vi "Grid_Create_Files_Headers.vi"(7 "resume":T1, 8 "Error in (no error)":errorcluster, 9 "Settings":T3={"Drift Correction Settings"={"Drift Correction every"=80, "Drift correction Pixels"=256, "Channel index (0-23)"=0, "MaxImagesBack"=2, "Threshold"=2, "Increment"=8, "max applied Drift Correction"=20, "Correct Drift"=TRUE, "Correlate"=0, "Correct z drift"=FALSE, "zdrift \nDuration (s)"=0.0}, "Spectroscopy Setting"={"Imaging Current"=1e-11, "ref Current"=7e-11, "tip Speed (m/s)"=2e-09, "Imaging Bias"=0.02, "ref Bias"=-0.1, "preSTS delay [ms]"=500, "STS z offset"=2e-10, "during Spec Bias (V)"=-0.1, "trigger1 < Hz"=0.0, "trigger 2 >Hz"=0.0, "autoStop"=FALSE, "Spectroscopy"=0, "PLL ON/OFF"=TRUE, "readjust setpoint every "=1, "z Reference"=FALSE, "Lock In"=TRUE}, "Misc"={"File name"="symmetric_node_zOff=200p", "Email when finished"="cornelius.krull@monash.edu,Dhaneesh.Gopalakrishnan@monash.edu,marina.castelli@monash.edu"}, "Grid Settings"={"type"=1, "type order"=1, "X pixel"=0, "Y pixel"=0, "Grid_Parms"={"center X (m)"=0.0, "center Y (m)"=0.0, "width (m)"=0.0, "height (m)"=0.0, "angle (deg)"=0.0}}} {"Grid Settings"."type order" items=["Line", "Grid"]; "Grid Settings"."type" items=["Line", "Grid"]; "Spectroscopy Setting"."Spectroscopy" items=["Bias", "zSpec"]; "Spectroscopy Setting"."trigger 2 >Hz" format="%#_6p"; "Spectroscopy Setting"."trigger1 < Hz" format="%#_6p"; "Spectroscopy Setting"."during Spec Bias (V)" format="%#_5p"; "Spectroscopy Setting"."STS z offset" format="%#_6p"; "Spectroscopy Setting"."ref Bias" format="%#_6p"; "Spectroscopy Setting"."Imaging Bias" format="%#_6p"; "Spectroscopy Setting"."tip Speed (m/s)" format="%.2p"; "Spectroscopy Setting"."ref Current" format="%#_6p"; "Spectroscopy Setting"."Imaging Current" format="%#_6p"; "Drift Correction Settings"."Correlate" items=["first Frame", "successive Frames"]; "Drift Correction Settings"."max applied Drift Correction" min=1 max=100 step=1 format="%.0p"; "Drift Correction Settings"."Threshold" min=1 step=1; "Drift Correction Settings"."Channel index (0-23)" items=["Current"=0, "Z (m)"=14]}, 11 "Application ref in":refnum<vi>) -> (0 "error out":errorcluster, 1 "topoFilePath":path, 2 "FileRefs":T2, 3 "Application ref out":refnum<vi>)   [LabVIEW 2014]
uses:
  <userlib>/Nanonis Prog Interface V5/Nanonis Prog Interface.lvlib
panel:
  in  "Attributes in":string[][](table)
  # "z Spectroscopy"
  # "GRID points"
  # "Increase this if no Drift was detected for \na certain number of images"
  # "% of image size"
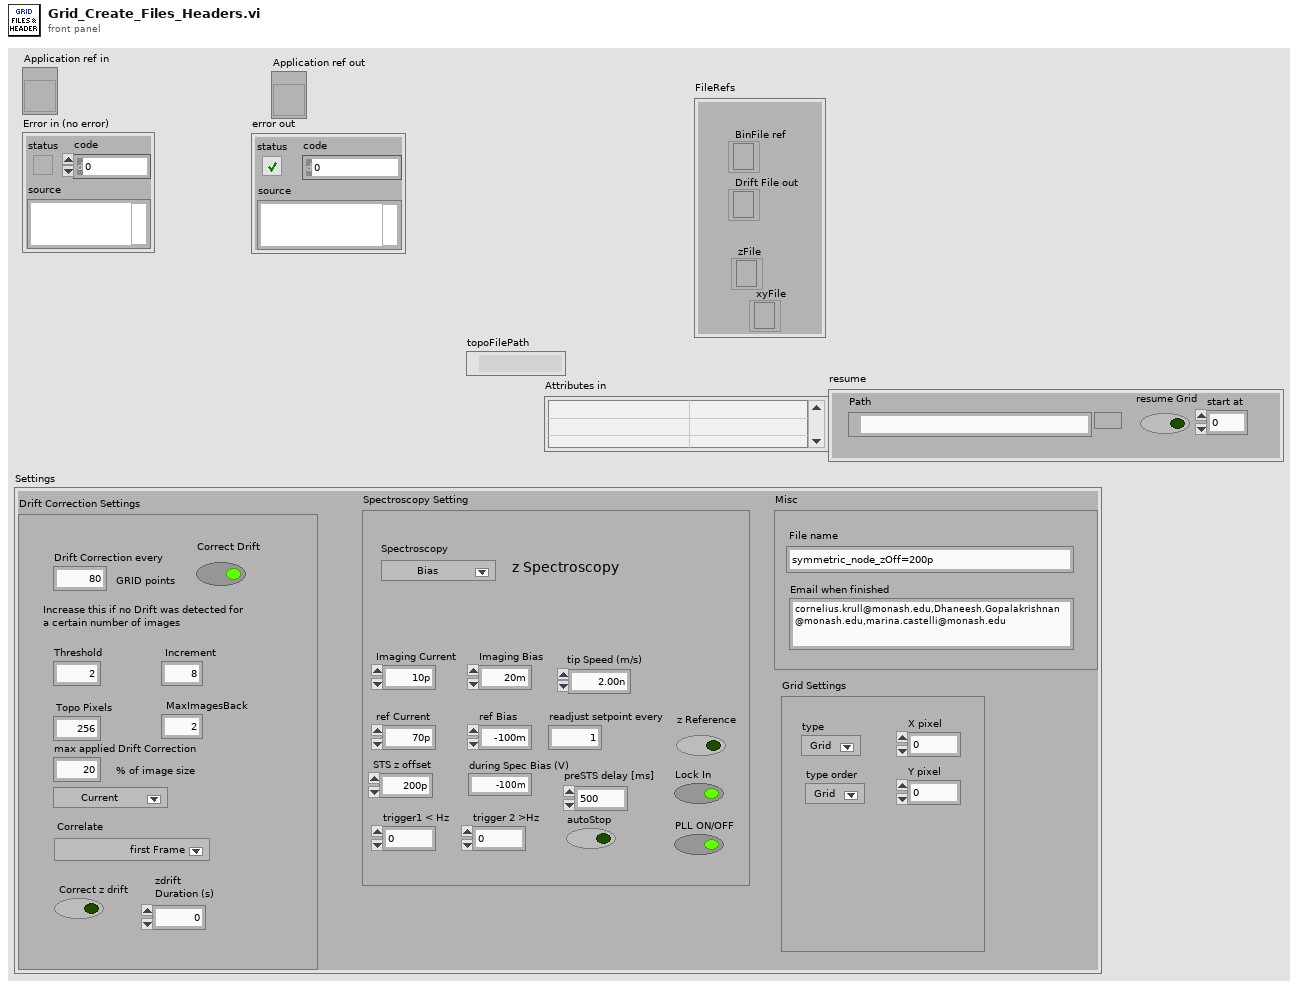
[diagram p1: front panel]
types:
  T1 = cluster{"resume Grid":bool, "Path":path, "start at":i32}
  T2 = cluster{"Drift File out":refnum<file>, "zFile":refnum<file>, "BinFile ref":refnum<file>, "xyFile":refnum<file>}
  T3 = cluster{"Drift Correction Settings":cluster{"Drift Correction every":i32, "Drift correction Pixels":i32, "Channel index (0-23)":u8, "MaxImagesBack":i32, "Threshold":i32, "Increment":i32, "max applied Drift Correction":i32, "Correct Drift":bool, "Correlate":u16, "Correct z drift":bool, "zdrift \nDuration (s)":dbl}, "Spectroscopy Setting":cluster{"Imaging Current":dbl, "ref Current":dbl, "tip Speed (m/s)":sgl, "Imaging Bias":dbl, "ref Bias":dbl, "preSTS delay [ms]":u32, "STS z offset":dbl, "during Spec Bias (V)":sgl, "trigger1 < Hz":sgl, "trigger 2 >Hz":sgl, "autoStop":bool, "Spectroscopy":u16, "PLL ON/OFF":bool, "readjust setpoint every ":i32, "z Reference":bool, "Lock In":bool}, "Misc":cluster{"File name":string, "Email when finished":string}, "Grid Settings":cluster{"type":u16, "type order":u16, "X pixel":i64, "Y pixel":i64, "Grid_Parms":cluster{"center X (m)":sgl, "center Y (m)":sgl, "width (m)":sgl, "height (m)":sgl, "angle (deg)":sgl}}}
  T4 = cluster{"Z averaging time (s)":sgl, "Z offset (m)":sgl, "Initial settling time (s)":sgl}
  T5 = enum16{"open", "replace", "create", "open or create", "replace or create", "replace or create with confirmation"}
  T6 = cluster{"center X (m)":sgl, "center Y (m)":sgl, "width (m)":sgl, "height (m)":sgl, "angle (deg)":sgl}
  T7 = cluster{"Max. slew rate (V/s)":sgl, "Settling time (s)":sgl, "Integration time (s)":sgl}
  T8 = cluster{"End settling time (s)":sgl, "Z control time (s)":sgl}
  T9 = cluster{"Z averaging time (s)":sgl, "Initial settling time (s)":sgl}
  T10 = cluster{"Max. slew rate (m/s)":sgl, "Settling time (s)":sgl, "Integration time (s)":sgl}
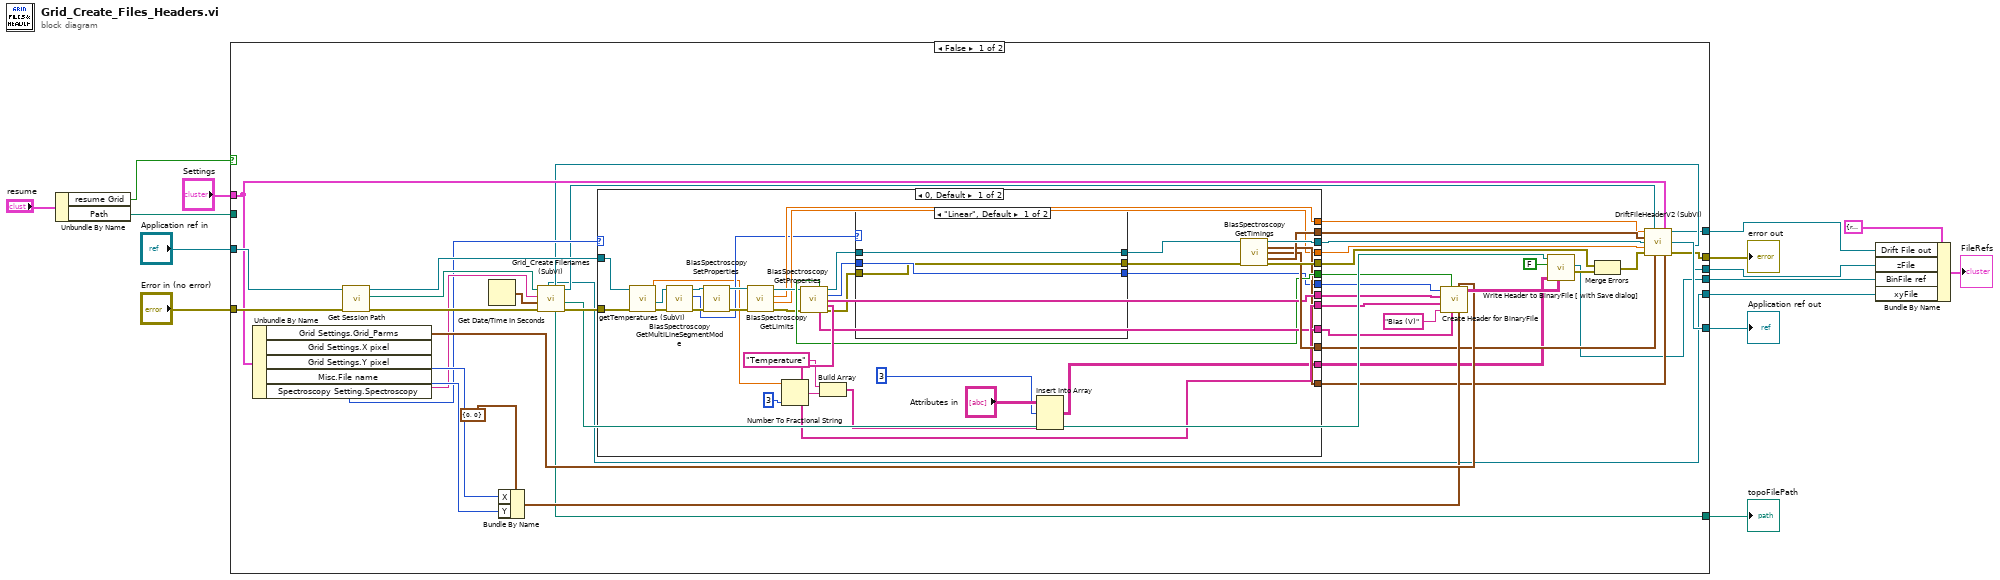
[diagram p0: block diagram]
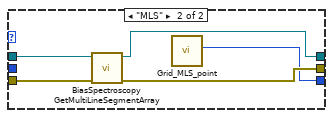
[diagram p2: hidden frame]
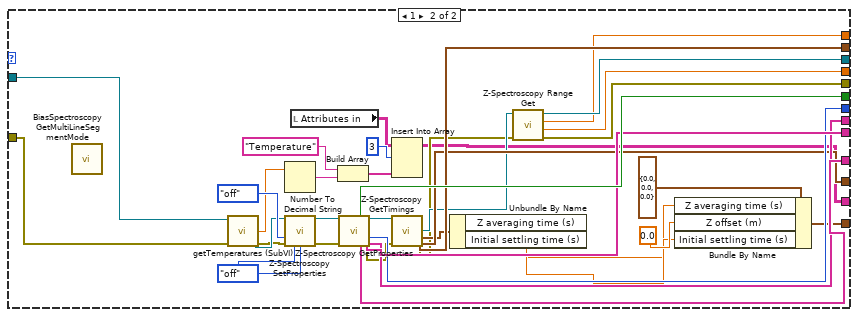
[diagram p3: hidden frame]
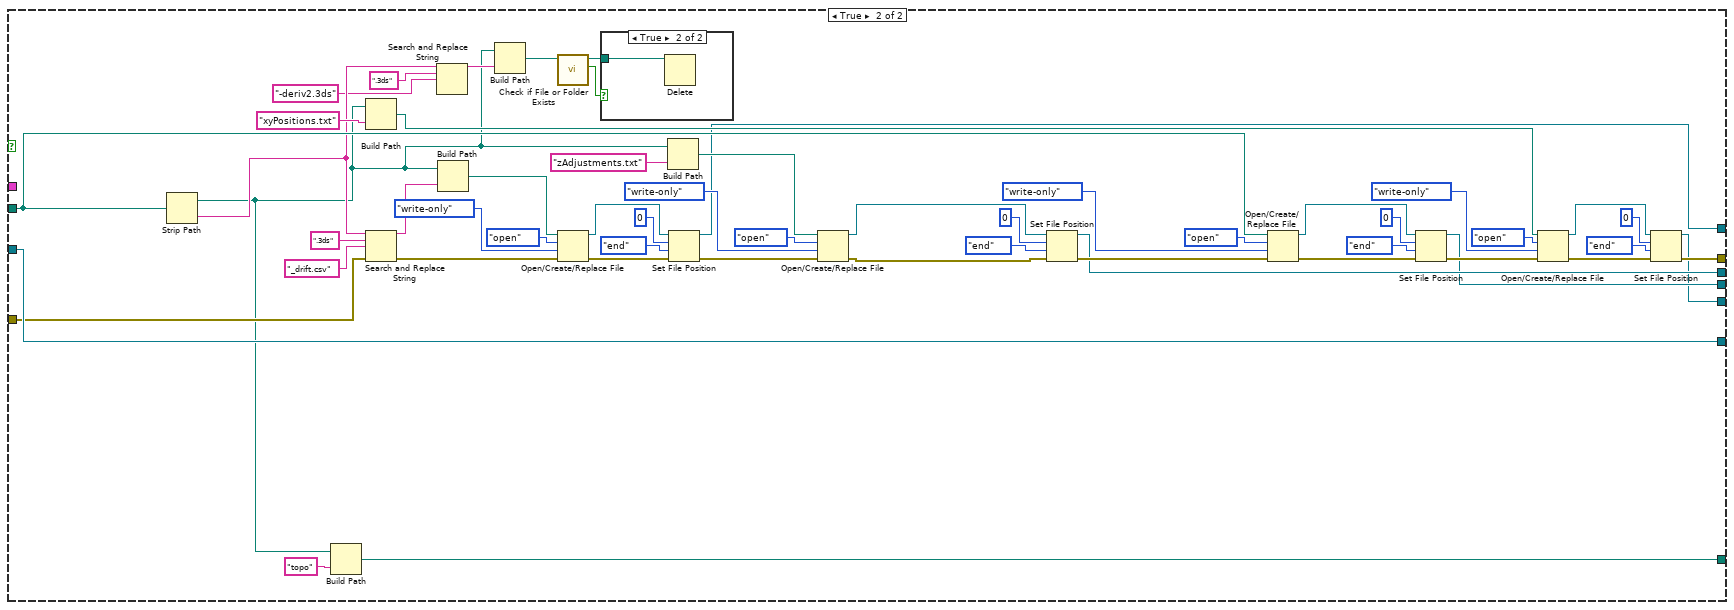
[diagram p4: hidden frame]
diagram:
  n1 = Unbundle By Name("resume") -> ("resume Grid"=w3:bool, "Path"=w1:path)
  n2 = case shown="False" w3 {
    tunnel: "Application ref in" -> [w56 w191]
    tunnel: "Error in (no error)" -> [w55 w170]
    tunnel: "Settings" -> [w32 _]
    tunnel: [w27 w191] -> w12
    tunnel: [w25 w153] -> w11
    tunnel: [w22 w149] -> w10
    tunnel: [w21 w150] -> w9
    tunnel: [w20 w159] -> w8
    tunnel: [w18 w146] -> w5
    tunnel: [w17 w186] -> w2
    tunnel: w1 -> [_ w188]
    frame False {
      n3 = Unbundle By Name(w32) -> ("Grid Settings.Grid_Parms"=w40:T6, "Grid Settings.X pixel"=w38:i64, "Grid Settings.Y pixel"=w37:i64, "Misc.File name"=w31:string, "Spectroscopy Setting.Spectroscopy"=w30:u16)
      n4 = call <userlib>:"Get Session Path.vi"("error in (no error)"=w55, "Application ref in"=w56) -> ("error out"=w53:errorcluster, "Session path"=w54:path, "Application ref out"=w52:refnum<vi>)  [unwired: 7 in]
      n5 = Get Date/Time In Seconds() -> (seconds since 1Jan1904=w19:timestamp)
      n6 = Bundle By Name(cluster=cluster{"X":i32, "Y":i32} {"X"=0, "Y"=0} ("Grid points"), "X"=w38, "Y"=w37) -> (w36:cluster{"X":i32, "Y":i32})
      n7 = call "Grid_Create Filenames (SubVI).vi"("error in (no error)"=w53, "seconds since 1Jan1904"=w19, "File name"=w31, "Session path"=w54) -> ("error out"=w57:errorcluster, "binFilePath"=w50:path, "Drift File out"=w29:refnum<file>, "topoFilePath"=w17:path, "zFile"=w21:refnum<file>, "xyFile"=w18:refnum<file>)  [unwired: 1 in, 1 out]
      n8 = case shown="0, Default" w30 {
        tunnel: [w86 w137] -> w41
        tunnel: [w88 w136] -> w44
        tunnel: [w92 w116] -> w47
        tunnel: [w87 w135] -> w45
        tunnel: [w75 w134] -> w42
        tunnel: [w89 w133] -> w43
        tunnel: w52 -> [w67 w112]
        tunnel: [w91 w131] -> w33
        tunnel: [w90 w130] -> w34
        tunnel: [w85 w119] -> w35
        tunnel: [w93 w117] -> w28
        tunnel: w57 -> [w69 w110]
        tunnel: [w80 w114] -> w24
        tunnel: [w79 w113] -> w23
        tunnel: [w62 w102] -> w16
        frame 0, Default {
          n9 = call "getTemperatures (SubVI).vi"("error in (no error)"=w69, "Application in"=w67) -> ("error out"=w68:errorcluster, "Application ref out"=w66:refnum<vi>, "TSTM"=w65:dbl)  [unwired: 6 in, 1 out]
          n10 = call <userlib>:"BiasSpectroscopy GetMultiLineSegmentMode.vi"("Error in (no error)"=w68, "Application ref in"=w66) -> ("Error out"=w77:errorcluster, "Sweep mode"=w74:enum16{"Linear", "MLS"}, "Application ref out"=w78:refnum<vi>)  [unwired: 5 in]
          n11 = call <userlib>:"BiasSpectroscopy SetProperties.vi"("Application ref in"=w78, "Error in (no error)"=w77) -> ("Application ref out"=w84:refnum<vi>, "Error out"=w81:errorcluster)  [unwired: 12 in]
          n12 = call <userlib>:"BiasSpectroscopy GetLimits.vi"("Error in (no error)"=w81, "Application ref in"=w84) -> ("Error out"=w82:errorcluster, "End value (V)"=w79:sgl, "Start value (V)"=w80:sgl, "Application ref out"=w83:refnum<vi>)  [unwired: 4 in]
          n13 = Number To Fractional String(number=w65, precision (6)=i16 3 ("width (-)")) -> (F-format string=w60:string)  [unwired: 2 in]
          n14 = call <userlib>:"BiasSpectroscopy GetProperties.vi"("Application ref in"=w83, "Error in (no error)"=w82) -> ("Backward sweep"=w86:bool, "Application ref out"=w73:refnum<vi>, "Number of points"=w76:i32, "Channels"=w89:string[], "Parameters"=w88:string[], "Fixed parameters"=w87:string[], "Error out"=w71:errorcluster)  [unwired: 5 in, 2 out]
          n15 = Build Array("Temperature" ("element"), w60) -> (w59:string[])
          n16 = case shown="\"Linear\", Default" w74 {
            tunnel: w76 -> [w96 _]
            tunnel: [w96 w97] -> w75
            tunnel: w73 -> [w94 w101]
            tunnel: [w94 w100] -> w72
            tunnel: w71 -> [w95 w99]
            tunnel: [w95 w98] -> w70
            frame "Linear", Default {
            }
            frame "MLS" {
              n17 = call <userlib>:"BiasSpectroscopy GetMultiLineSegmentArray.vi"("Error in (no error)"=w99, "Application ref in"=w101) -> ("Error out"=w98:errorcluster, "Application ref out"=w100:refnum<vi>)  [unwired: 5 in, 1 out]
              n18 = call "Grid_MLS_point.vi"() -> ("points"=w97:i32)  [unwired: 11 in]
            }
          }
          n19 = Insert Into Array(array="Attributes in", index (row)=3, new element=w59) -> (w62:string[][])  [unwired: 1 in]
          n20 = call <userlib>:"BiasSpectroscopy GetTimings.vi"("Application ref in"=w72, "Error in (no error)"=w70) -> ("Application ref out"=w93:refnum<vi>, "Initialization"=w85:T4, "Sweep Timing"=w90:T7, "End of Sweep"=w91:T8, "Error out"=w92:errorcluster)  [unwired: 9 in]
        }
        frame 1 {
          w129 = enum16{"no change", "on", "off"}."off" ("Save dialog")
          n21 = call <userlib>:"BiasSpectroscopy GetMultiLineSegmentMode.vi"() -> ()  [unwired: 7 in, 3 out]
          n22 = call "getTemperatures (SubVI).vi"("error in (no error)"=w110, "Application in"=w112) -> ("error out"=w109:errorcluster, "Application ref out"=w111:refnum<vi>, "TSTM"=w104:dbl)  [unwired: 6 in, 1 out]
          n23 = Number To Decimal String(number=w104) -> (decimal integer string=w107:string)  [unwired: 1 in]
          n24 = call <userlib>:"Z-Spectroscopy SetProperties.vi"("Application ref in"=w111, "Autosave"=enum16{"no change", "on", "off"}."off" ("Autosave (no change)"), "error in (no error)"=w109, "Save dialog"=w129, "Save all sweeps (no change)"=w129) -> ("Application ref out"=w127:refnum<vi>, "error out"=w126:errorcluster)  [unwired: 9 in]
          n25 = local read "Attributes in"() -> (w103:string[][])
          n26 = Build Array("Temperature" ("element"), w107) -> (w108:string[])
          n27 = call <userlib>:"Z-Spectroscopy GetProperties.vi"("Application ref in"=w127, "error in (no error)"=w126) -> ("Backward sweep"=w137:bool, "Application ref out"=w132:refnum<vi>, "Number of points"=w134:i32, "Channels"=w133:string[], "Parameters"=w136:string[], "Fixed parameters"=w135:string[], "error out"=w125:errorcluster)  [unwired: 6 in, 1 out]
          n28 = Insert Into Array(array=w103, index (row)=3, new element=w108) -> (w102:string[][])  [unwired: 1 in]
          n29 = call <userlib>:"Z-Spectroscopy GetTimings.vi"("Application ref in"=w132, "Error in (no error)"=w125) -> ("Application ref out"=w118:refnum<vi>, "Initialization"=w120:T9, "Sweep Timing"=w130:T10, "End of Sweep"=w131:T8, "Error out"=w115:errorcluster)  [unwired: 9 in]
          n30 = Unbundle By Name(w120) -> ("Z averaging time (s)"=w122:sgl, "Initial settling time (s)"=w123:sgl)
          n31 = call <userlib>:"Z-Spectroscopy Range Get.vi"("error in (no error)"=w115, "Application ref in"=w118) -> ("error out"=w116:errorcluster, "Z distance (m)"=w113:sgl, "Z offset (m)"=w114:sgl, "Application ref out"=w117:refnum<vi>)  [unwired: 5 in]
          n32 = Bundle By Name(cluster=T4 {"Z averaging time (s)"=0.0, "Z offset (m)"=0.0, "Initial settling time (s)"=0.0} ("Initialization"), "Z averaging time (s)"=w122, "Z offset (m)"=sgl 0.0, "Initial settling time (s)"=w123) -> (w119:T4)
        }
      }
      n33 = call <userlib>:"Create Header for BinaryFile.vi"("Grid points"=w36, "Grid param"=w40, "Fixed parameters"=w45, "Backward sweep"=w41, "Sweep signal"="Bias (V)" ("Sweep Signal"), "Parameters"=w44, "Channels"=w43, "Points per sweep"=w42) -> ("Header (fixed attributes)"=w51:string[][])  [unwired: 3 in]
      n34 = call <userlib>:"Write Header to BinaryFile [ with Save dialog].vi"("Fixed Attributes"=w51, "Attributes in"=w16, "Show Dialog? (T)"=FALSE, "Filename"=w50) -> ("Error out"=w48:errorcluster, "File ref"=w22:refnum<file>)  [unwired: 4 in, 2 out]
      n35 = Merge Errors(w47, w48) -> (w26:errorcluster)
      n36 = call "DriftFileHeaderV2 (SubVI).vi"("Start value (V)"=w24, "Byte Stream File in"=w29, "Settings"=w32, "End of Sweep"=w33, "Application ref in"=w28, "End value (V)"=w23, "error in (no error)"=w26, "Sweep Timing"=w34, "Initialization"=w35) -> ("Byte Stream File out"=w20:refnum<file>, "Application ref out"=w27:refnum<vi>, "error out"=w25:errorcluster)  [unwired: 4 in]
    }
    frame True {
      n37 = Strip Path(path=w188) -> (stripped path=w165:path, name=w169:string)
      n38 = Build Path(base path=w165, name or relative path="topo") -> (appended path=w186:path)
      n39 = Build Path(base path=w165, name or relative path="xyPositions.txt") -> (appended path=w174:path)
      n40 = Search and Replace String(input string=w169, search string=".3ds", replace string="_drift.csv" ("replace string (\"\")"), error in=w170) -> (result string=w183:string, error out=w171:errorcluster)  [unwired: 4 in, 2 out]
      n41 = Search and Replace String(input string=w169, search string=".3ds", replace string="-deriv2.3ds" ("replace string (\"\")")) -> (result string=w166:string)  [unwired: 5 in, 3 out]
      n42 = Build Path(base path=w165, name or relative path=w183) -> (appended path=w180:path)
      n43 = Build Path(base path=w165, name or relative path=w166) -> (appended path=w164:path)
      n44 = call <vilib>:"Check if File or Folder Exists.vi"("path"=w164) -> ("file or folder exists?"=w163:bool, "dup path"=w162:path)  [unwired: 8 in, 1 out]
      n45 = Open/Create/Replace File(file path (use dialog)=w180, error in=w171, operation (0:open)=T5."open", access (0:read/write)=enum16{"read/write", "read-only", "write-only"}."write-only") -> (refnum out=w158:refnum<file>, error out=w161:errorcluster)  [unwired: 2 in, 1 out]
      n46 = case shown="True" w163 {
        tunnel: w162 -> [_ w192]
        frame False {
        }
        frame True {
          n47 = Delete(path (use dialog)=w192) -> ()  [unwired: 4 in, 3 out]
        }
      }
      n48 = Build Path(base path=w165, name or relative path="zAdjustments.txt") -> (appended path=w173:path)
      n49 = Set File Position(offset (in bytes) (0)=i64 0, refnum=w158, from (0:start)=enum16{"start", "end", "current"}."end", error in=w161) -> (refnum out=w159:refnum<file>, error out=w160:errorcluster)
      n50 = Open/Create/Replace File(file path (use dialog)=w173, error in=w160, operation (0:open)=T5."open", access (0:read/write)=enum16{"read/write", "read-only", "write-only"}."write-only") -> (refnum out=w151:refnum<file>, error out=w157:errorcluster)  [unwired: 2 in, 1 out]
      n51 = Set File Position(offset (in bytes) (0)=i64 0, refnum=w151, from (0:start)=enum16{"start", "end", "current"}."end", error in=w157) -> (refnum out=w150:refnum<file>, error out=w156:errorcluster)
      n52 = Open/Create/Replace File(file path (use dialog)=w188, error in=w156, operation (0:open)=T5."open", access (0:read/write)=enum16{"read/write", "read-only", "write-only"}."write-only") -> (refnum out=w148:refnum<file>, error out=w155:errorcluster)  [unwired: 2 in, 1 out]
      n53 = Set File Position(offset (in bytes) (0)=i64 0, refnum=w148, from (0:start)=enum16{"start", "end", "current"}."end", error in=w155) -> (refnum out=w149:refnum<file>, error out=w154:errorcluster)
      n54 = Open/Create/Replace File(file path (use dialog)=w174, error in=w154, operation (0:open)=T5."open", access (0:read/write)=enum16{"read/write", "read-only", "write-only"}."write-only") -> (refnum out=w147:refnum<file>, error out=w152:errorcluster)  [unwired: 2 in, 1 out]
      n55 = Set File Position(offset (in bytes) (0)=i64 0, refnum=w147, from (0:start)=enum16{"start", "end", "current"}."end", error in=w152) -> (refnum out=w146:refnum<file>, error out=w153:errorcluster)
    }
  }
  "Application ref out" <- w12
  "error out" <- w11
  "topoFilePath" <- w2
  n56 = Bundle By Name(cluster=T2 {"Drift File out"=refnum, "zFile"=refnum, "BinFile ref"=refnum, "xyFile"=refnum} ("FileRefs"), "Drift File out"=w8, "zFile"=w9, "BinFile ref"=w10, "xyFile"=w5) -> (→"FileRefs":T2)
